vi "AVL SLIN.vi"(8 "error in (no error)":errorcluster caption="Fehler (Eingang, kein Fehler)") -> (0 "error out":errorcluster caption="Fehler (Ausgang)")   [LabVIEW 2020, in "Linearisierung v2.lvlib" / "Gasteiler.lvlib"]
uses:
  Gasteiler.lvlib
  AK-Komm Gasteiler/Aktionen AK Komm.ctl
  AK-Komm Gasteiler/AK Komm Gasteiler.lvlib
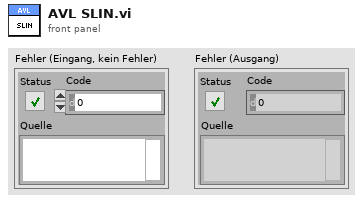
[diagram p1: front panel]
types:
  T1 = typedef "Linearisierung v2.lvlib/Gasteiler.lvlib/AK Komm Gasteiler.lvlib/Aktionen AK Komm.ctl" = enum16{"lesen", "initialisieren", "beenden", "Status", "SMAN", "SREM", "STBY", "ASTF", "ASTZ", "SLST", "AGAT", "EGAK", "AGAK", "AKAK", "ADRU", "SKOP", "SVSA", "SVSZ", "SONO", "SAIR", "SNOX", "ANOX", "SSPL", "SRUC", "SLIN", "ALST", "ETYP", "SVIO", "LCYL", "CCYL", "DCYL", "SCYL", "GCYL", "DRGV", "DRDC"}
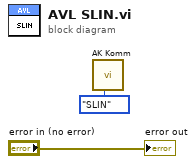
[diagram p0: block diagram]
diagram:
  n1 = call "AK Komm.vi"("Aktionen"=Aktionen_AK_Komm."SLIN") -> ()  [unwired: 4 in, 7 out]
  "error out" <- "error in (no error)"
